vi "S2DS_ConfigWriteAdditionalInfo (SubVI).vi"(8 "error in (no error)":errorcluster, 10 "False channel":string[][](array[string]), 11 "Refnum in":T1) -> (0 "error out":errorcluster, 3 "Refnum out":T1)   [LabVIEW 2025]
uses:
  <vilib>/Utility/config.llb/Config Data RefNum.ctl
  <vilib>/Utility/config.llb/Write Key (I32).vi
  <vilib>/Utility/config.llb/Write Key (String).vi
  <vilib>/Utility/config.llb/NI_LVConfig.lvlib
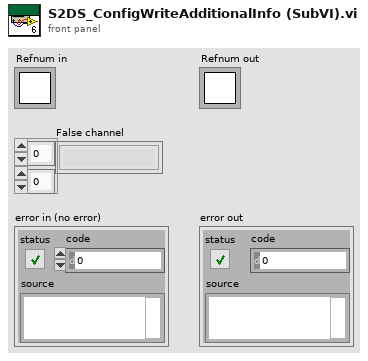
[diagram p1: front panel]
types:
  T1 = typedef "NI_LVConfig.lvlib/Config Data RefNum.ctl" = refnum<k1>
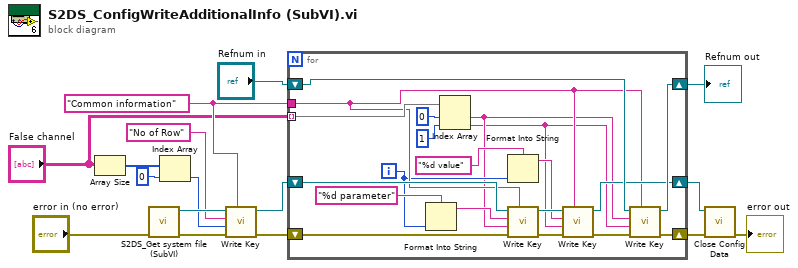
[diagram p0: block diagram]
diagram:
  w11 = "Common information" ("section")
  n1 = Array Size(array="False channel") -> (size(s)=w8:i32[])
  n2 = call "S2DS_Get system file (SubVI).vi"("error in (no error)"="error in (no error)") -> ("error out"=w13:errorcluster, "Refnum out"=w12:T1)  [unwired: 9 in]
  n3 = Index Array(array=w8, index=0) -> (element=w6:i32)
  n4 = call-poly <vilib>:"Write Key.vi"("section"=w11, "error in (no error)"=w13, "value"=w6, "key"="No of Row", "refnum"=w12) -> ("error out"=w3:errorcluster, "refnum out"=w5:T1)  [unwired: 4 in, 1 out]
  n5 = for {
    tunnel: "False channel" -> [w36] mode=indexing
    shift-right: [w32] -> w15
    shift-left: "Refnum in" -> [w33]
    shift-right: [w31] -> w2
    shift-left: w3 -> [w18]
    tunnel: w11 -> [w26]
    shift-right: [w27] -> w4
    shift-left: w5 -> [w30]
    i -> [w23]
    n6 = Format Into String(format string="%d parameter", w23) -> (resulting string=w24:string)  [unwired: 2 in, 1 out]
    n7 = Index Array(array=w36, index #1=0 ("index"), index #2=1 ("index")) -> (element #1=w20:string, element #2=w19:string)
    n8 = Format Into String(format string="%d value", w23) -> (resulting string=w21:string)  [unwired: 2 in, 1 out]
    n9 = call-poly <vilib>:"Write Key.vi"("section"=w26, "error in (no error)"=w18, "value"=w20, "key"=w24, "refnum"=w30) -> ("error out"=w29:errorcluster, "refnum out"=w28:T1)  [unwired: 4 in, 1 out]
    n10 = call-poly <vilib>:"Write Key.vi"("section"=w26, "error in (no error)"=w29, "value"=w19, "key"=w21, "refnum"=w28) -> ("error out"=w17:errorcluster, "refnum out"=w27:T1)  [unwired: 4 in, 1 out]
    n11 = call-poly <vilib>:"Write Key.vi"("section"=w26, "error in (no error)"=w17, "value"=w19, "key"=w20, "refnum"=w33) -> ("error out"=w31:errorcluster, "refnum out"=w32:T1)  [unwired: 4 in, 1 out]
  }
  "Refnum out" <- w15
  n12 = call <vilib>:"Close Config Data.vi"("error in (no error)"=w2, "refnum"=w4) -> ("error out"=→"error out":errorcluster)  [unwired: 8 in, 1 out]
